vi "p42m comms viewer.vi"() -> ()   [LabVIEW 2018]
uses:
  <vilib>/nican/nican.llb/CanFrameTimed.ctl
panel:
  out "Array":cluster{bool, timestamp, "Data":u8[]}[](array[cluster]) {"?" format="%<%.3X>T"; "Data" format="%x"}
  out "data":T2(array[cluster]) {"TX Msgs"."Data" format="%.0x"; "TX Msgs"."ArbitrationId" format="%.0x"; "TX Msgs"."Timestamp" format="%<%I:%M:%S%3u %p\n%m/%d/%Y>T"; "RX Msgs"."Data" format="%.0x"; "RX Msgs"."ArbitrationId" format="%.0x"; "RX Msgs"."Timestamp" format="%<%I:%M:%S%3u %p\n%m/%d/%Y>T"}
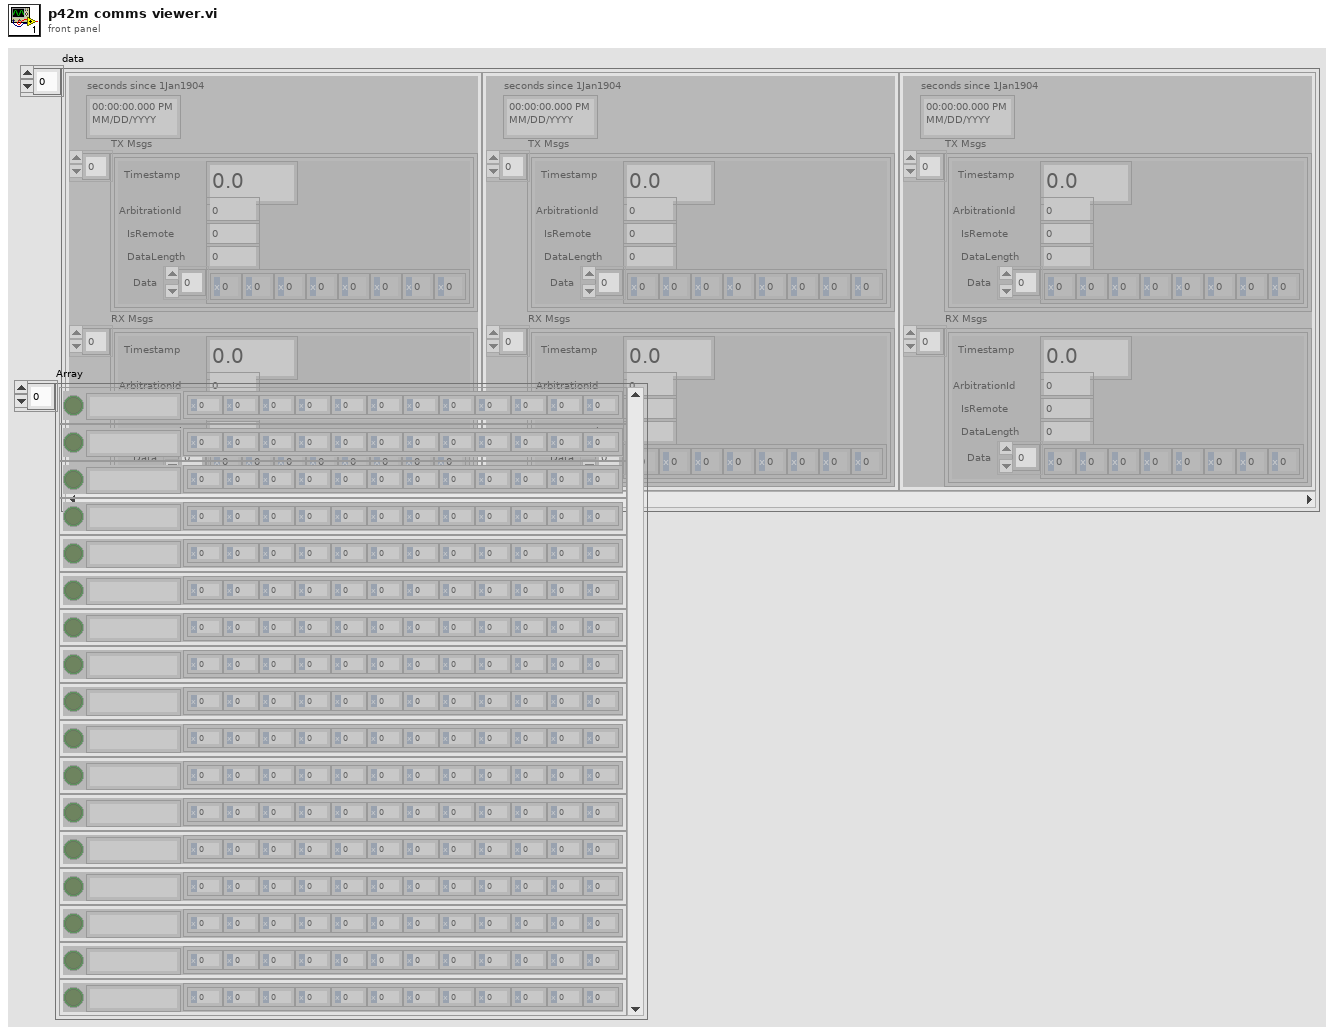
[diagram p1: front panel]
types:
  T1 = typedef "CanFrameTimed.ctl" = cluster{"Timestamp":dbl, "ArbitrationId":u32, "IsRemote":u8, "DataLength":u8, "Data":u8[]}
  T2 = cluster{"seconds since 1Jan1904":timestamp, "TX Msgs":T1[], "RX Msgs":T1[]}[]
  T3 = cluster{"seconds since 1Jan1904":timestamp, "TX Msgs":T1[], "RX Msgs":T1[]}
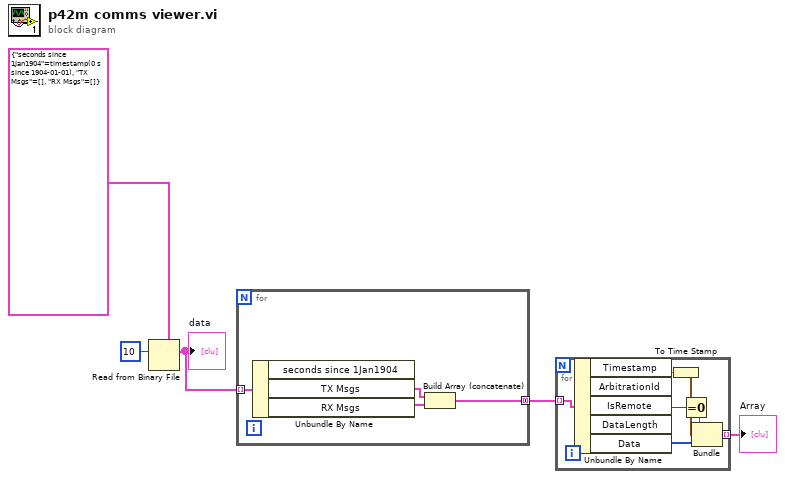
[diagram p0: block diagram]
diagram:
  n1 = Read from Binary File(5:T3 {"seconds since 1Jan1904"=timestamp(0 s since 1904-01-01), "TX Msgs"=[], "RX Msgs"=[]} ("output cluster"), 10:10 ("count (1)")) -> (2:w3:T2)  [unwired: 4 in, 3 out]
  "data" <- w3
  n2 = for {
    tunnel: w3 -> [w9] mode=indexing
    tunnel: [w6] -> w2 mode=concatenating
    n3 = Unbundle By Name(w9) -> ("TX Msgs"=w8:T1[], "RX Msgs"=w7:T1[])  [unwired: 1 out]
    n4 = Build Array (concatenate)(w8, w7) -> (w6:T1[])
  }
  n5 = for {
    tunnel: w2 -> [w16] mode=indexing
    tunnel: [w10] -> w1 mode=indexing
    n6 = Unbundle By Name(w16) -> ("Timestamp"=w13:dbl, "IsRemote"=w15:u8, "Data"=w11:u8[])  [unwired: 2 out]
    n7 = To Time Stamp(1:w13) -> (0:w12:timestamp)
    n8 = Equal To 0?(x=w15) -> (x = 0?=w14:bool)
    n9 = Bundle(w14, w12, "Data"=w11) -> (w10:cluster{bool, timestamp, "Data":u8[]})  [unwired: 1 in]
  }
  "Array" <- w1
